vi "Pop (DBL).vi"(10 "Key":string, 11 "Dictionary in":variant) -> (1 "Value":dbl, 2 "found":bool, 3 "Dictionary out":variant)   [LabVIEW 2013, in "Dictionary.lvlib"]
doc: "Pop (Remove and return) value from dictionary with passed in key."
uses:
  Dictionary.lvlib
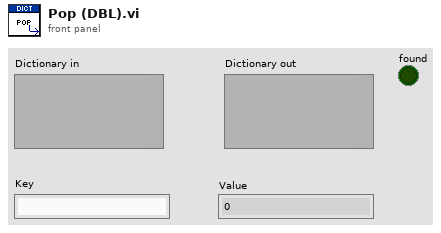
[diagram p1: front panel]
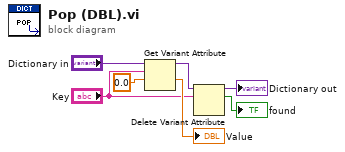
[diagram p0: block diagram]
diagram:
  n1 = Get Variant Attribute(Variant="Dictionary in", name="Key", default value (empty Variant)=0.0) -> (duplicate Variant=w6:variant, value=→"Value":dbl)  [unwired: 1 in, 2 out]
  n2 = Delete Variant Attribute(6:"Key", 7:w6) -> (2:→"found":bool, 3:→"Dictionary out":variant)  [unwired: 1 in, 1 out]
